vi "MPExxx_get_modulation_information.vi"(0 "VISA session":refnum<visa-resource-name>, 1 "error in (no error)":errorcluster) -> (2 "dup VISA session":refnum<visa-resource-name>, 3 "Select Output to Modulate":i8(ring) items=["None", "Voltage", "Current"], 4 "Modulation Type":u16(ring) items=["Multiplication", "Addition"], 5 "error out":errorcluster)   [LabVIEW 2012]
doc: "This VI form returns the mode of modulation and modulation type."
uses:
  MPExxx Globals.gbl
panel:
  # "MAGNA-POWER"
  # "Electronics"
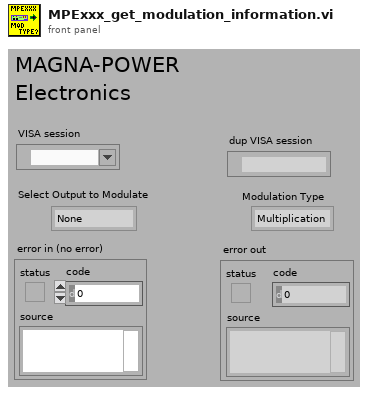
[diagram p1: front panel]
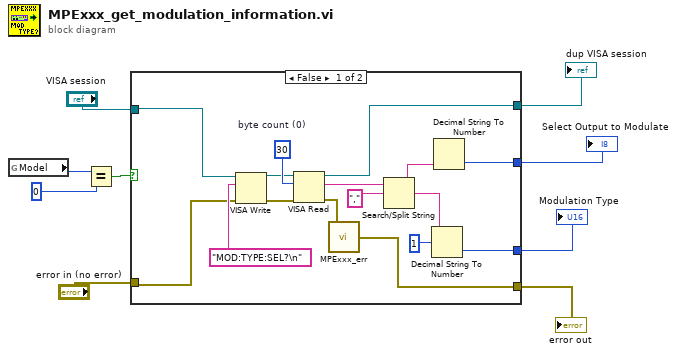
[diagram p0: block diagram]
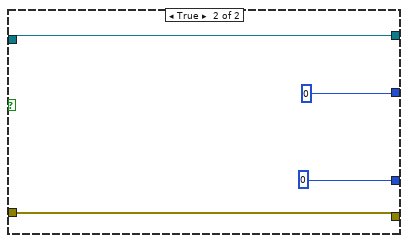
[diagram p2: hidden frame]
diagram:
  n1 = global read "MPExxx Globals.gbl" "Model"() -> (w7:u8)
  n2 = Equal?(x=w7, y=0) -> (x = y?=w9:bool)
  n3 = case shown="False" w9 {
    tunnel: "VISA session" -> [w15 w29]
    tunnel: "error in (no error)" -> [w14 w28]
    tunnel: [w13 w29] -> w4
    tunnel: [w12 w28] -> w3
    tunnel: [w11 0] -> w2
    tunnel: [w10 0] -> w1
    frame False {
      w19 = u32 30  # byte count (0)
      n4 = VISA Write(VISA resource name=w15, write buffer="MOD:TYPE:SEL?\n", error in (no error)=w14) -> (VISA resource name out=w18:refnum<visa-resource-name>, error out=w17:errorcluster)  [unwired: 1 out]
      n5 = VISA Read(VISA resource name=w18, byte count=w19, error in (no error)=w17) -> (VISA resource name out=w13:refnum<visa-resource-name>, read buffer=w25:string, error out=w20:errorcluster)  [unwired: 1 out]
      n6 = call "MPExxx_err.vi"("error in (no error)"=w20) -> ("error out"=w12:errorcluster)
      n7 = Search/Split String(string=w25, search string/char (-)=",") -> (substring before match=w22:string, match + rest of string=w23:string)  [unwired: 1 in, 1 out]
      n8 = Decimal String To Number(string=w23, offset=1) -> (number=w11:i32)  [unwired: 1 in, 1 out]
      n9 = Decimal String To Number(string=w22) -> (number=w10:i32)  [unwired: 2 in, 1 out]
    }
    frame True {
    }
  }
  "error out" <- w3
  "dup VISA session" <- w4
  "Select Output to Modulate" <- w1
  "Modulation Type" <- w2
